vi "Vertical and Horizontal Digitizer Configuration.vi"(7 "Channel(s)":T1[](array[typedef]), 8 "error in (no error)":errorcluster, 11 "PXIe5105 in":refnum<class "PXIe5105.lvclass">) -> (0 "error out":errorcluster, 3 "PXIe5105 out":refnum<class "PXIe5105.lvclass">)   [LabVIEW 2018, in "PXIe5105.lvlib" / "PXIe5105.lvclass"]
uses:
  PXIe5105.lvclass
  PPLs/Oscilloscope/Parent/Oscilloscope.lvlibp/Custom Controls/Analog Channels.ctl
  PXIe5105.lvclass/PXIe5105.ctl
  PPLs/Oscilloscope/Parent/Oscilloscope.lvlibp
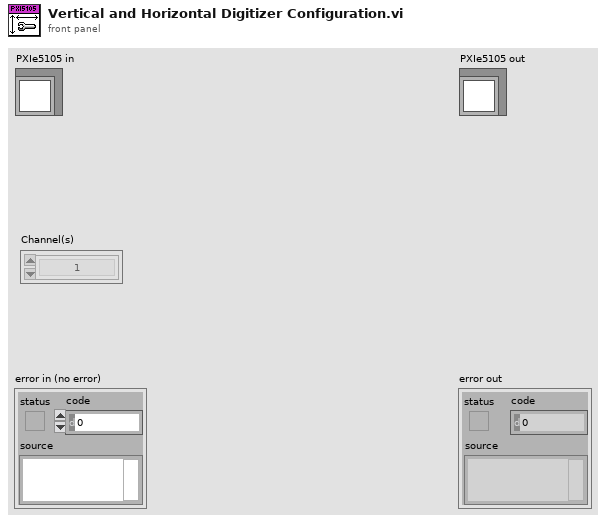
[diagram p1: front panel]
types:
  T1 = typedef "Oscilloscope.lvlibp/Analog Channels.ctl" = enum16{"1", "2", "3", "4", "5", "6", "7", "8", "9", "10", "11", "12", "13", "14", "15", "16"}
  T2 = typedef "niScope vertical coupling.ctl" = i32
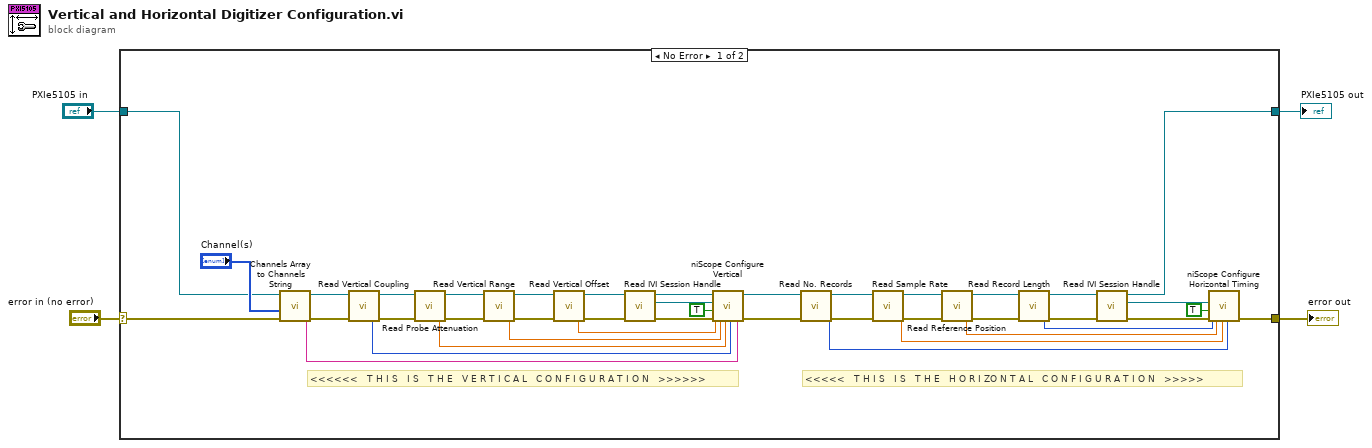
[diagram p0: block diagram]
diagram:
  n1 = case shown="No Error" "error in (no error)" {
    selector: "error in (no error)" -> [w39 w46]
    tunnel: [w44 w46] -> w3
    tunnel: [w11 w45] -> w1
    tunnel: "PXIe5105 in" -> [w40 w45]
    frame No Error {
      # "<<<<<   T H I S   I S   T H E   H O R I ZO N T A L   C O N F I G U R A T I O N   >>>>>"
      # "<<<<<<   T H I S   I S   T H E   V E R T I C A L   C O N F I G U R A T I O N   >>>>>>"
      n2 = call "Channels Array to Channels String.vi"("error in (no error)"=w39, "Channel(s) Array"="Channel(s)", "PXIe5105 in"=w40) -> ("error out"=w43:errorcluster, "Channels String"=w24:string, "PXIe5105 out"=w41:refnum<class "PXIe5105.lvclass">)  [unwired: 6 in]
      n3 = call "Read Vertical Coupling.vi"("error in (no error)"=w43, "PXIe5105 in"=w41) -> ("error out"=w36:errorcluster, "vertical coupling"=w25:T2, "PXIe5105 out"=w33:refnum<class "PXIe5105.lvclass">)  [unwired: 7 in]
      n4 = call "Read Probe Attenuation.vi"("error in (no error)"=w36, "PXIe5105 in"=w33) -> ("error out"=w37:errorcluster, "Probe Attenuation"=w26:dbl, "PXIe5105 out"=w34:refnum<class "PXIe5105.lvclass">)  [unwired: 7 in]
      n5 = call "Read Vertical Range.vi"("error in (no error)"=w37, "PXIe5105 in"=w34) -> ("error out"=w38:errorcluster, "Vertical Range"=w27:dbl, "PXIe5105 out"=w35:refnum<class "PXIe5105.lvclass">)  [unwired: 7 in]
      n6 = call "Read Vertical Offset.vi"("error in (no error)"=w38, "PXIe5105 in"=w35) -> ("error out"=w31:errorcluster, "Vertical Offset"=w28:dbl, "PXIe5105 out"=w32:refnum<class "PXIe5105.lvclass">)  [unwired: 7 in]
      n7 = call "Read IVI Session Handle.vi"("error in (no error)"=w31, "PXIe5105 in"=w32) -> ("error out"=w30:errorcluster, "IVI Session Handle"=w29:refnum<k15>, "PXIe5105 out"=w14:refnum<class "PXIe5105.lvclass">)  [unwired: 7 in]
      n8 = call <instrlib>:"niScope Configure Vertical.vi"("instrument handle"=w29, "probe attenuation"=w26, "vertical coupling"=w25, "channels"=w24, "vertical range"=w27, "vertical offset"=w28, "error in"=w30, "channel enabled"=TRUE) -> ("error out"=w13:errorcluster)  [unwired: 6 in, 1 out]
      n9 = call "Read No. Records.vi"("error in (no error)"=w13, "PXIe5105 in"=w14) -> ("error out"=w22:errorcluster, "No. Records"=w6:i32, "PXIe5105 out"=w19:refnum<class "PXIe5105.lvclass">)  [unwired: 7 in]
      n10 = call "Read Sample Rate.vi"("error in (no error)"=w22, "PXIe5105 in"=w19) -> ("error out"=w21:errorcluster, "Sample Rate"=w7:dbl, "PXIe5105 out"=w18:refnum<class "PXIe5105.lvclass">)  [unwired: 7 in]
      n11 = call "Read Reference Position.vi"("error in (no error)"=w21, "PXIe5105 in"=w18) -> ("error out"=w20:errorcluster, "Reference Position"=w8:dbl, "PXIe5105 out"=w17:refnum<class "PXIe5105.lvclass">)  [unwired: 7 in]
      n12 = call "Read Record Length.vi"("error in (no error)"=w20, "PXIe5105 in"=w17) -> ("error out"=w16:errorcluster, "Record Length"=w9:i32, "PXIe5105 out"=w15:refnum<class "PXIe5105.lvclass">)  [unwired: 7 in]
      n13 = call "Read IVI Session Handle.vi"("error in (no error)"=w16, "PXIe5105 in"=w15) -> ("error out"=w12:errorcluster, "IVI Session Handle"=w10:refnum<k15>, "PXIe5105 out"=w11:refnum<class "PXIe5105.lvclass">)  [unwired: 7 in]
      n14 = call <instrlib>:"niScope Configure Horizontal Timing.vi"("instrument handle"=w10, "number of records"=w6, "enforce realtime"=TRUE, "min sample rate"=w7, "reference position"=w8, "error in"=w12, "min record length"=w9) -> ("error out"=w44:errorcluster)  [unwired: 7 in, 1 out]
    }
    frame Error {
    }
  }
  "error out" <- w3
  "PXIe5105 out" <- w1
